vi "配置初始化.vi"(8 "error in (no error)":errorcluster caption="错误输入（无错误）") -> (0 "error out":errorcluster)   [LabVIEW 2016, in "环境动力监测库.lvlib"]
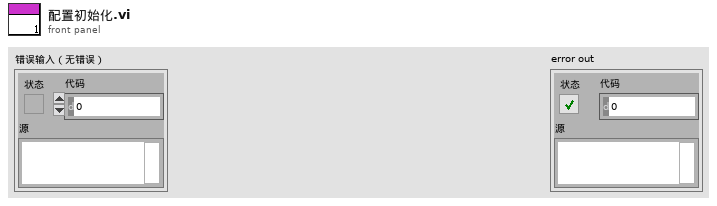
[diagram p1: front panel]
types:
  T1 = cluster{"市电监测":bool, "用水量监测":bool, "烟雾监测":bool, "温度湿度":bool, "振动监测":bool, "红外入侵监测":bool, "漏水监测":bool, "门禁开关监测":bool, "门禁开关监测2":bool, "视频监测":bool, "UPS监测":bool, "空调监测":bool, "冰箱监测":bool, "排气扇监测":bool, "蓄电池监测":bool, "蓄电池监测2":bool, "GPS监测":bool, "北斗监测":bool, "气象监测":bool, "智能门禁监测":bool, "废液监测":bool, "废液监测2":bool, "灭火装置监测":bool}
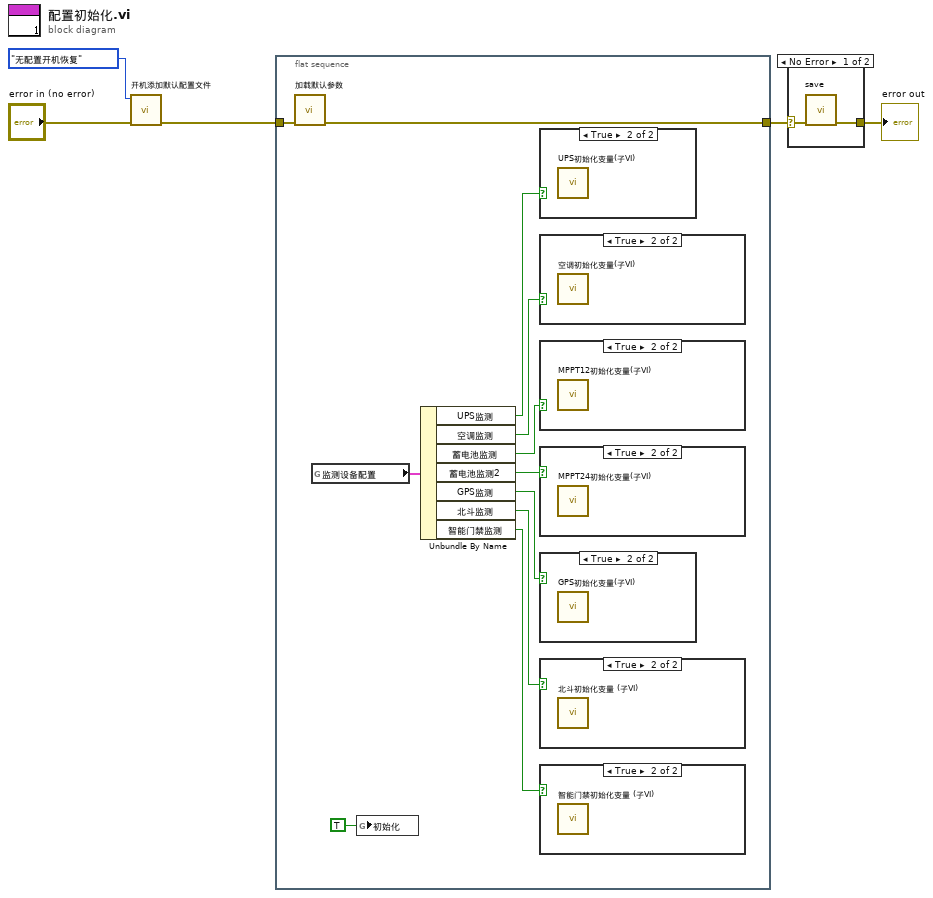
[diagram p0: block diagram]
diagram:
  n1 = call "开机添加默认配置文件.vi"("error in (no error)"="error in (no error)", "恢复默认方式"=enum16{"无配置开机恢复", "手动恢复"}."无配置开机恢复") -> ("error out"=w3:errorcluster)  [unwired: 9 in]
  n2 = flat-sequence {
    tunnel: [w7] -> w2
    tunnel: w3 -> [w8]
    frame #0 {
      n3 = call "加载默认参数.vi"("error IO"=w8) -> ("error IO 2"=w7:errorcluster)  [unwired: 10 in]
      n4 = global read "断电保存全局变量.vi" "监测设备配置"() -> (w16:T1)
      n5 = global write "外部交互全局变量.vi" "初始化"(TRUE ("初始化")) -> ()
      n6 = Unbundle By Name(w16) -> ("UPS监测"=w15:bool, "空调监测"=w14:bool, "蓄电池监测"=w13:bool, "蓄电池监测2"=w12:bool, "GPS监测"=w11:bool, "北斗监测"=w10:bool, "智能门禁监测"=w9:bool)
      n7 = case shown="True" w15 {
        frame False {
        }
        frame True {
          n8 = call "UPS初始化变量(子VI).vi"() -> ()  [unwired: 11 in, 1 out]
        }
      }
      n9 = case shown="True" w14 {
        frame False {
        }
        frame True {
          n10 = call "空调初始化变量(子VI).vi"() -> ()  [unwired: 11 in, 1 out]
        }
      }
      n11 = case shown="True" w13 {
        frame False {
        }
        frame True {
          n12 = call "MPPT12初始化变量(子VI).vi"() -> ()  [unwired: 11 in, 1 out]
        }
      }
      n13 = case shown="True" w12 {
        frame False {
        }
        frame True {
          n14 = call "MPPT24初始化变量(子VI).vi"() -> ()  [unwired: 11 in, 1 out]
        }
      }
      n15 = case shown="True" w11 {
        frame False {
        }
        frame True {
          n16 = call "GPS初始化变量(子VI).vi"() -> ()  [unwired: 11 in, 1 out]
        }
      }
      n17 = case shown="True" w10 {
        frame False {
        }
        frame True {
          n18 = call "北斗初始化变量 (子VI).vi"() -> ()  [unwired: 11 in, 1 out]
        }
      }
      n19 = case shown="True" w9 {
        frame False {
        }
        frame True {
          n20 = call "智能门禁初始化变量 (子VI).vi"() -> ()  [unwired: 11 in, 1 out]
        }
      }
    }
  }
  n21 = case shown="No Error" w2 {
    selector: w2 -> [w18 w19]
    tunnel: [w17 w19] -> w1
    frame No Error {
      n22 = call "save.vi"("error in (no error)"=w18) -> ("error out"=w17:errorcluster)  [unwired: 10 in]
    }
    frame Error {
    }
  }
  "error out" <- w1
